vi "bodyTest.vi"(7 "LabVIEW Web Service Request":refnum<class "Web Request.lvclass">, 9 "unit":dbl, 10 "nominalPressure":dbl caption="pressure" format="%#g", 11 "time":dbl format="%#g") -> (2 "value":string, 3 "actualPressure":dbl)   [LabVIEW 2015]
uses:
  <vilib>/wsapi/Web Request.lvclass
  <vilib>/Waveform/WDTOps.llb/WDT Append Waveforms DBL.vi
panel:
  in  "Stop (Pressure Reading)":bool
  out "startingPressure":dbl format="%#_2g"
  in  "Start timer":bool
  out "data":waveform(dbl)[](graph)
  out "timer":dbl
  in  "Stop timer":bool
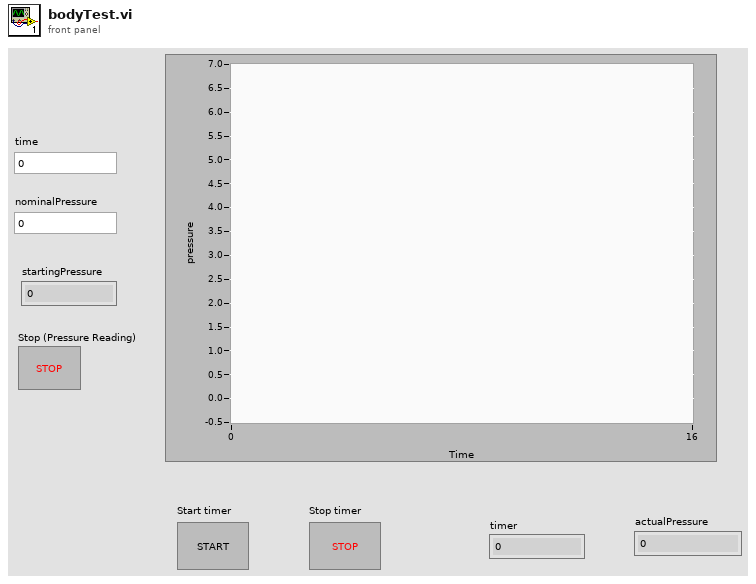
[diagram p1: front panel]
types:
  T1 = typedef "imagedata.ctl" = cluster{"image type":i32, "image depth":i32, "image":u8[], "mask":u8[], "colors":u32[], "Rectangle":cluster{"left":i16, "top":i16, "right":i16, "bottom":i16}}
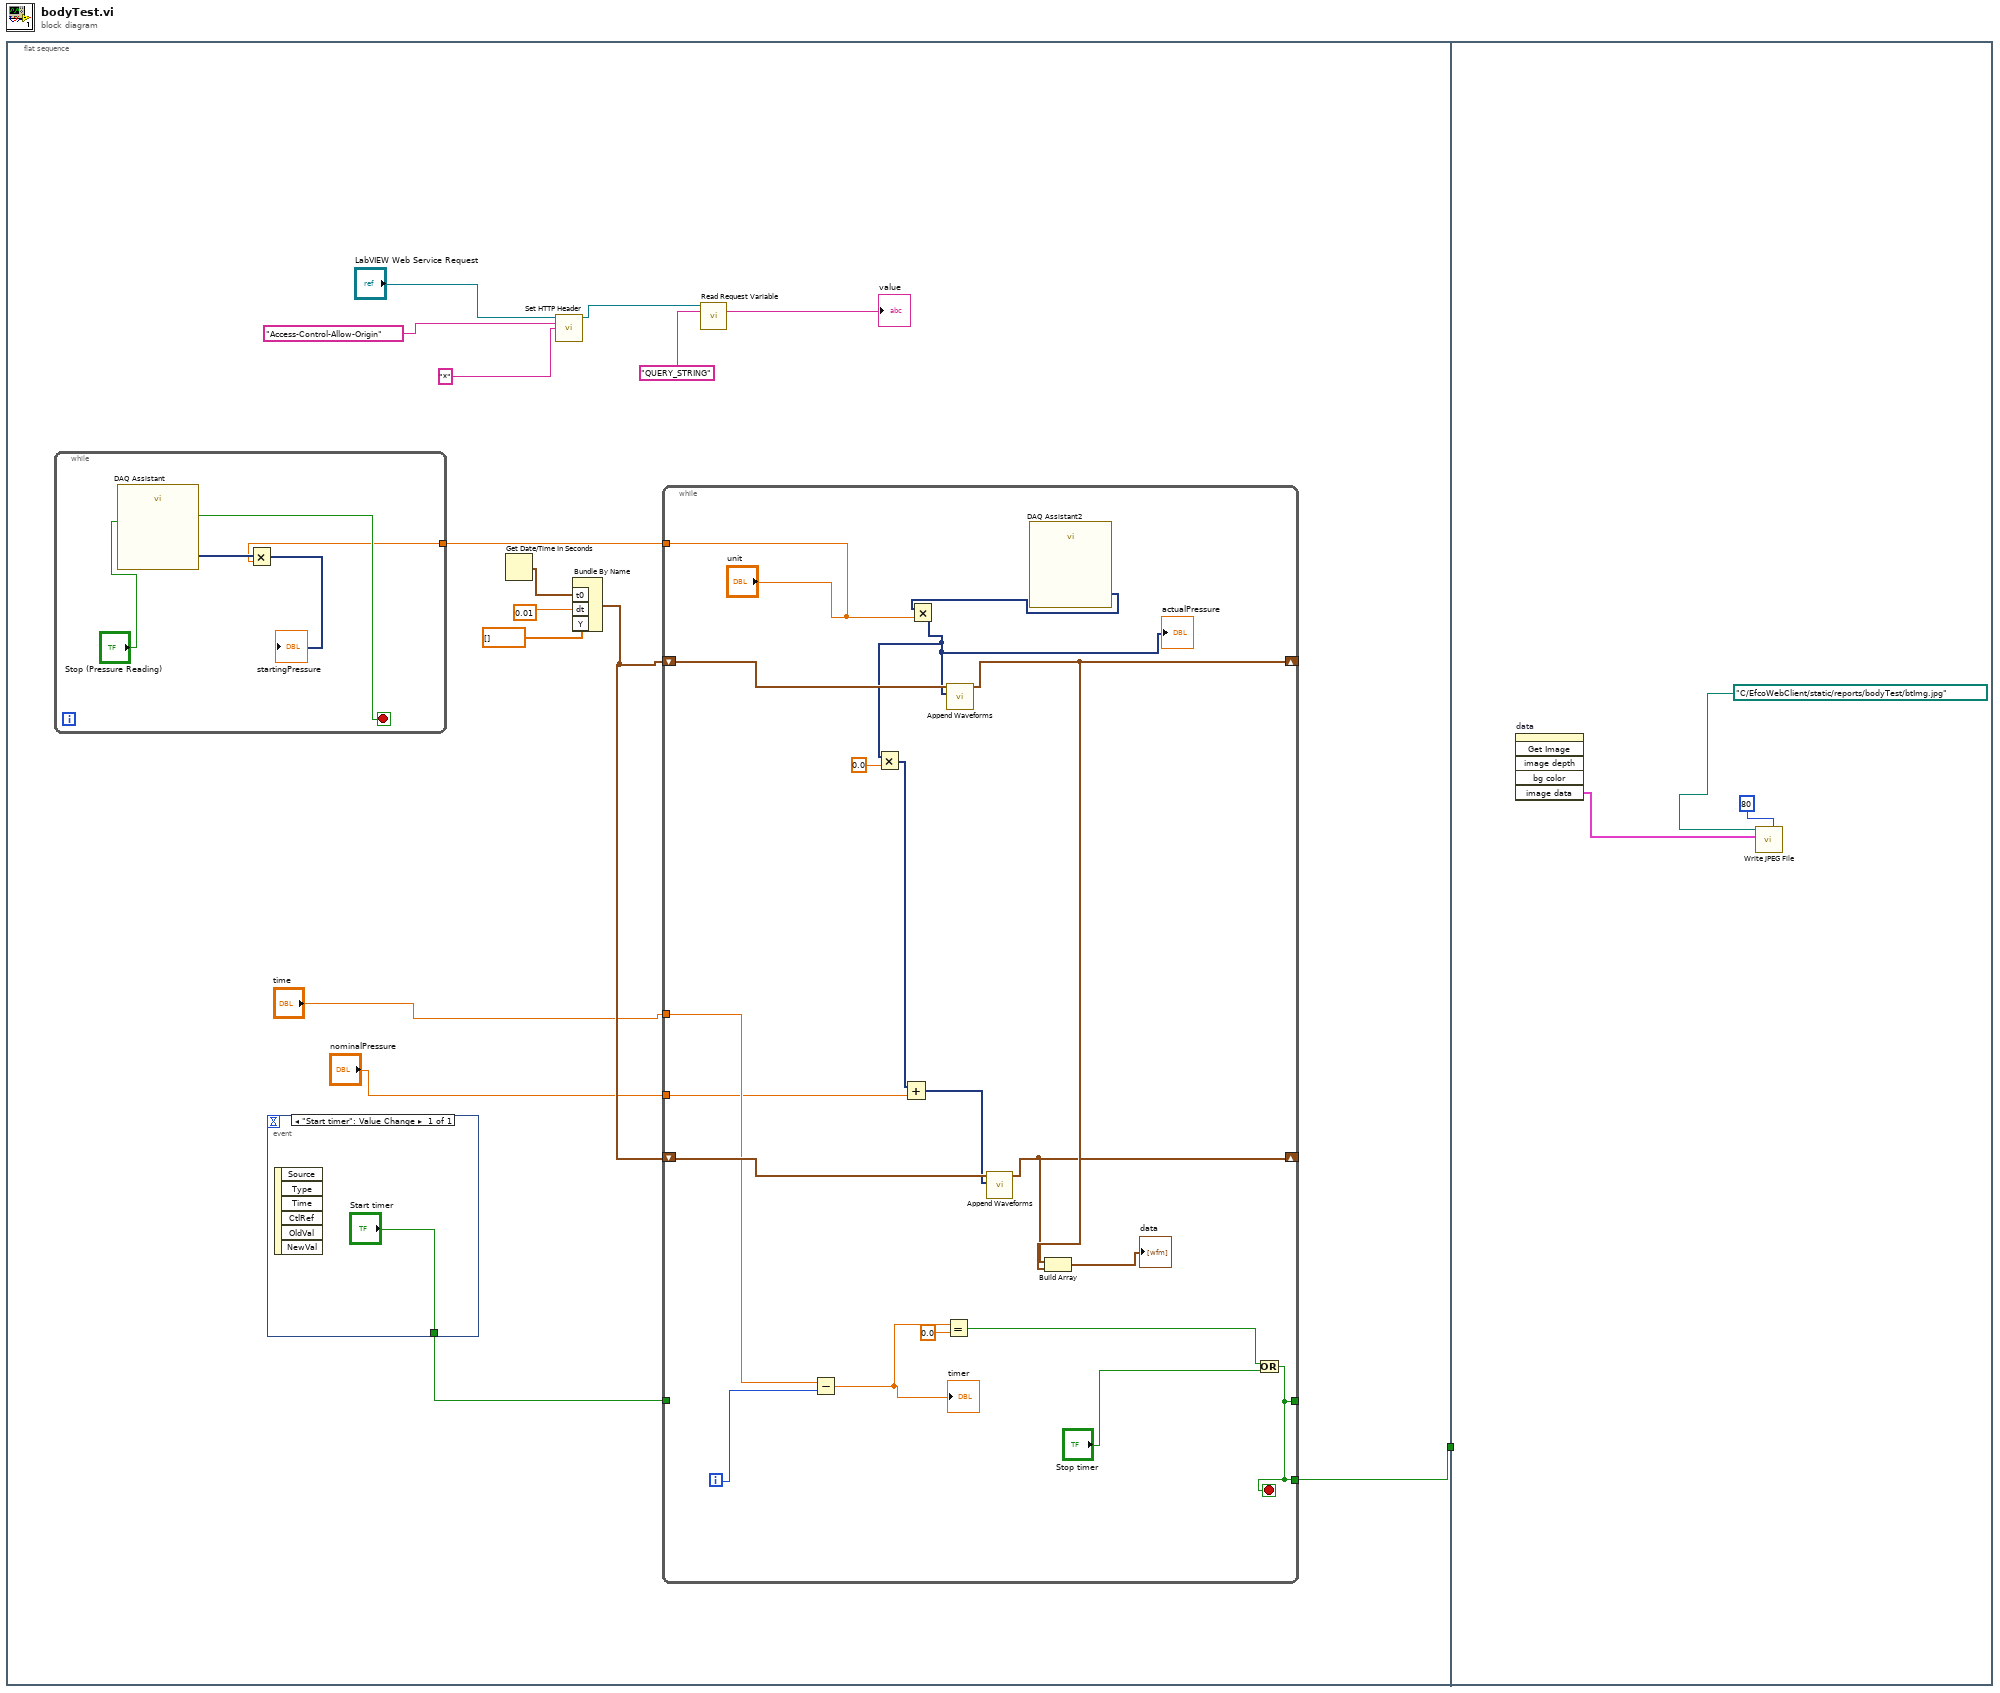
[diagram p0: block diagram]
diagram:
  n1 = flat-sequence {
    tunnel: [w9] -> w1
    tunnel: w1 -> [_]
    frame #0 {
      n2 = event shown="[0] \"Start timer\": Value Change" {
        selector: _ -> [_]
        dyn-events: _ -> [_]
        timeout: _ -> [_]
        tunnel: ["Start timer"] -> w13
        event "Start timer": Value Change {
          n3 = event-data() -> ()  [unwired: 1 in, 6 out]
        }
      }
      n4 = Get Date/Time In Seconds() -> (seconds since 1Jan1904=w16:timestamp)
      n5 = call <vilib>:"Set HTTP Header.vi"("LabVIEW Web Service Request"="LabVIEW Web Service Request", "header"="Access-Control-Allow-Origin", "header value"="*") -> ("LabVIEW Web Service Request out"=w5:refnum<class "Web Request.lvclass">)  [unwired: 11 in, 1 out]
      n6 = Bundle By Name("t0"=w16, "dt"=0.01, "Y"=dbl[] []) -> (w12:waveform(dbl))  [unwired: 1 in]
      n7 = while {
        shift-right: [w37] -> _
        shift-left: w12 -> [w41]
        tunnel: "time" -> [w32]
        shift-right: [w36] -> _
        shift-left: w12 -> [w40]
        tunnel: w13 -> [_]
        tunnel: "nominalPressure" -> [w26]
        tunnel: [w25] -> _
        tunnel: [w25] -> w9
        tunnel: ["unit"] -> w2
        i -> [w33]
        stop <- w25 stop-if-true
        n8 = Subtract(x=w32, y=w33) -> (x-y=w31:dbl)
        "timer" <- w31
        n9 = Equal?(x=w31, y=0.0) -> (x = y?=w29:bool)
        n10 = call "DAQ Assistant2"() -> ("data"=w35:dynamicdata)  [unwired: 16 in, 3 out]
        n11 = Multiply(x=w35, y="unit") -> (x*y=w23:dynamicdata)
        "actualPressure" <- w23
        n12 = Multiply(x=w23, y=0.0) -> (x*y=w38:dynamicdata)
        n13 = Add(x=w38, y=w26) -> (x+y=w27:dynamicdata)
        n14 = call-poly <vilib>:"Append Waveforms.vi"("waveform B"=w23, "waveform A"=w41) -> ("waveform out"=w37:waveform(dbl))  [unwired: 8 in, 1 out]
        n15 = call-poly <vilib>:"Append Waveforms.vi"("waveform B"=w27, "waveform A"=w40) -> ("waveform out"=w36:waveform(dbl))  [unwired: 8 in, 1 out]
        n16 = Build Array(w36, w37) -> (→"data":waveform(dbl)[])
        n17 = Or(x=w29, y="Stop timer") -> (x .or. y?=w25:bool)
      }
      n18 = while {
        tunnel: w2 -> [w17]
        stop <- w18 stop-if-true
        n19 = call "DAQ Assistant"("stop (F)"="Stop (Pressure Reading)") -> ("data"=w21:dynamicdata, "stopped"=w18:bool)  [unwired: 15 in, 2 out]
        n20 = Multiply(x=w21, y=w17) -> (x*y=→"startingPressure":dynamicdata)
      }
      n21 = call <vilib>:"Read Request Variable.vi"("LabVIEW Web Service Request"=w5, "variable name"="QUERY_STRING") -> ("value"=→"value":string)  [unwired: 11 in, 2 out]
    }
    frame #1 {
      n22 = invoke on="data" class="WFGraph (strict)" method="Get Image"() -> ("image data"=w42:T1)  [unwired: 6 in, 5 out]
      n23 = call <vilib>:"Write JPEG File.vi"("quality (80)"=80, "image data"=w42, "path to JPEG file"=path "C:/EfcoWebClient/static/reports/bodyTest/btImg.jpg") -> ()  [unwired: 7 in, 2 out]
    }
  }
